vi "TPS System Start.vi"   [LabVIEW 2009]
doc: "This Vi starts up the full (or partial) set of VI necessary to operate the the Target Polarization System. The user should press the button that does reflects their wish. The control is set up for cases where the entire TPS system is moved to another disk or machine."
uses:
  TPS Global.vi
  <vilib>/Utility/config.llb/NI_LVConfig.lvlib
panel:
  # "Close Me!"
types:
  T1 = typedef "NI_LVConfig.lvlib/Config Data RefNum.ctl" = refnum<k1>
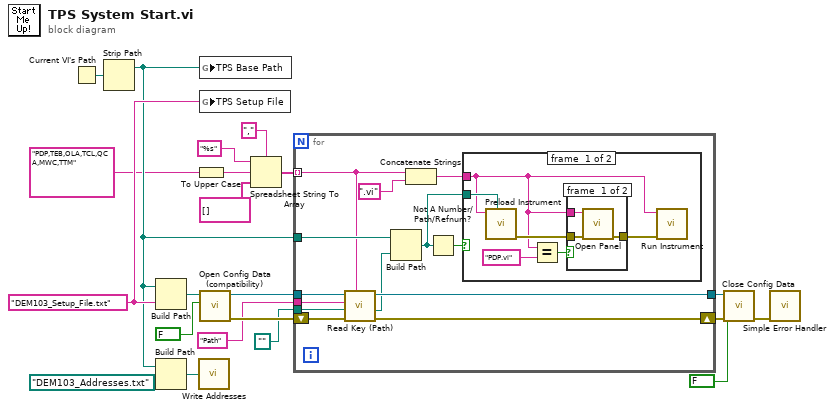
[diagram p0: block diagram]
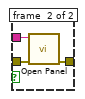
[diagram p2: hidden frame]
diagram:
  w8 = "DEM103_Setup_File.txt" ("TPS Setup File")
  n1 = Current VI's Path() -> (path=w10:path)
  n2 = Strip Path(path=w10) -> (stripped path=w4:path)  [unwired: 1 out]
  n3 = Build Path(base path=w4, name or relative path=w8) -> (appended path=w9:path)
  n4 = Build Path(base path=w4, name or relative path=path "DEM103_Addresses.txt") -> (appended path=w3:path)
  n5 = To Upper Case(1:"PDP,TEB,OLA,TCL,QCA,MWC,TTM") -> (0:w6:string)
  n6 = call "Write Addresses.vi"("Address File"=w3) -> ()
  n7 = global write "TPS Global.vi" "TPS Base Path"(w4) -> ()
  n8 = global write "TPS Global.vi" "TPS Setup File"(w8) -> ()
  n9 = call <vilib>:"Open Config Data (compatibility).vi"("create file if necessary (T)"=FALSE ("create file if necessary? (T)"), "configuration file path"=w9) -> ("error out"=w20:errorcluster, "refnum"=w19:T1)  [unwired: 7 in, 1 out]
  n10 = Spreadsheet String To Array(delimiter (Tab)=",", format string="%s", spreadsheet string=w6, array type (2D Dbl)=string[] [] ("Array Constant")) -> (array=w13:string[])
  n11 = for {
    shift-right: [w32] -> w17
    shift-left: w20 -> [w33]
    tunnel: w19 -> [w34]
    tunnel: [w31] -> w18
    tunnel: w13 -> [w26] mode=indexing
    tunnel: "Path" ("key") -> [w30]
    tunnel: path "" -> [w29]
    tunnel: w4 -> [w28]
    n12 = call <vilib>:"Read Key (Path).vi"("section"=w26, "error in (no error)"=w33, "default value"=w29, "key"=w30, "refnum"=w34) -> ("error out"=w32:errorcluster, "value"=w27:path, "refnum out"=w31:T1)  [unwired: 3 in, 1 out]
    n13 = Build Path(base path=w28, name or relative path=w27) -> (appended path=w23:path)
    n14 = Concatenate Strings(w26, ".vi" ("Substring")) -> (w24:string)
    n15 = Not A Number/Path/Refnum?(number/path/refnum=w23) -> (NaN/Path/Refnum?=w22:bool)
    n16 = case shown="False" w22 {
      tunnel: w24 -> [w36 _]
      tunnel: w23 -> [w38 _]
      frame #0 {
        n17 = call <vilib>:"Preload Instrument.vi"("VI path"=w38, "VI name"=w36) -> ("error out"=w39:errorcluster)  [unwired: 9 in]
        n18 = Equal?(x=w36, y="PDP.vi") -> (x = y?=w37:bool)
        n19 = case shown="False" w37 {
          tunnel: [w43 w46] -> w40
          tunnel: w39 -> [w42 w45]
          tunnel: w36 -> [w41 w44]
          frame #0 {
            n20 = call <vilib>:"Open Panel.vi"("error in (no error)"=w42, "VI name"=w41) -> ("error out"=w43:errorcluster)  [unwired: 9 in]
          }
          frame #1 {
            n21 = call <vilib>:"Open Panel.vi"("error in (no error)"=w45, "VI name"=w44) -> ("error out"=w46:errorcluster)  [unwired: 9 in]
          }
        }
        n22 = call <vilib>:"Run Instrument.vi"("error in (no error)"=w40, "VI name"=w36) -> ()  [unwired: 9 in, 1 out]
      }
      frame #1 {
      }
    }
  }
  n23 = call <vilib>:"Close Config Data.vi"("error in (no error)"=w17, "write file if changed (T)"=FALSE, "refnum"=w18) -> ("error out"=w7:errorcluster)  [unwired: 7 in, 1 out]
  n24 = call <vilib>:"Simple Error Handler.vi"("error in (no error)"=w7) -> ()  [unwired: 4 in, 5 out]
